vi "多参数断电保存全局变量.vi"() -> ()   [LabVIEW 2016, in "斯坦道原位多参数.lvlib"]
panel:
  in  "波特率":u32(ring)=115200 items=["9600"=9600, "19200"=19200, "115200"=115200]
  in  "传感器参数自动获取":bool=TRUE
  out "传感器参数modbus":u16[](array[numeric])
  in  "标样测试组数":dbl=1.0 caption="标样测试组数:"
  in  "水样测试组数":dbl=1.0 caption="水样测试组数:"
  in  "转刷清洗时间":dbl=30.0 caption="转刷清洗时间:"
  in  "上电初始化时间":dbl=5.0 caption="上电初始化时间:"
  in  "水样稳定时间":dbl=5.0 caption="水样稳定时间:"
  in  "ORP参数":T1
  in  "藻密度参数":T1
  in  "叶绿素参数":T1
  in  "浊度参数":T1
  in  "电导率参数":T1
  in  "溶解氧参数":T1
  in  "PH参数":T1
  in  "水温参数":T1
  in  "VISA Resource":refnum<visa-resource-name>="COM6"
  in  "运行周期":T2
  in  "质控参数设置":T3
  # "组"
  # "min"
  # "组"
  # "s"
  # "s"
  # "运行模式："
  # "质控参数设置"
  # "监测参数"
  # "水温"
  # "酸碱度"
  # "溶解氧"
  # "电导率"
  # "浊度"
  # "标样核查标准液浓度"
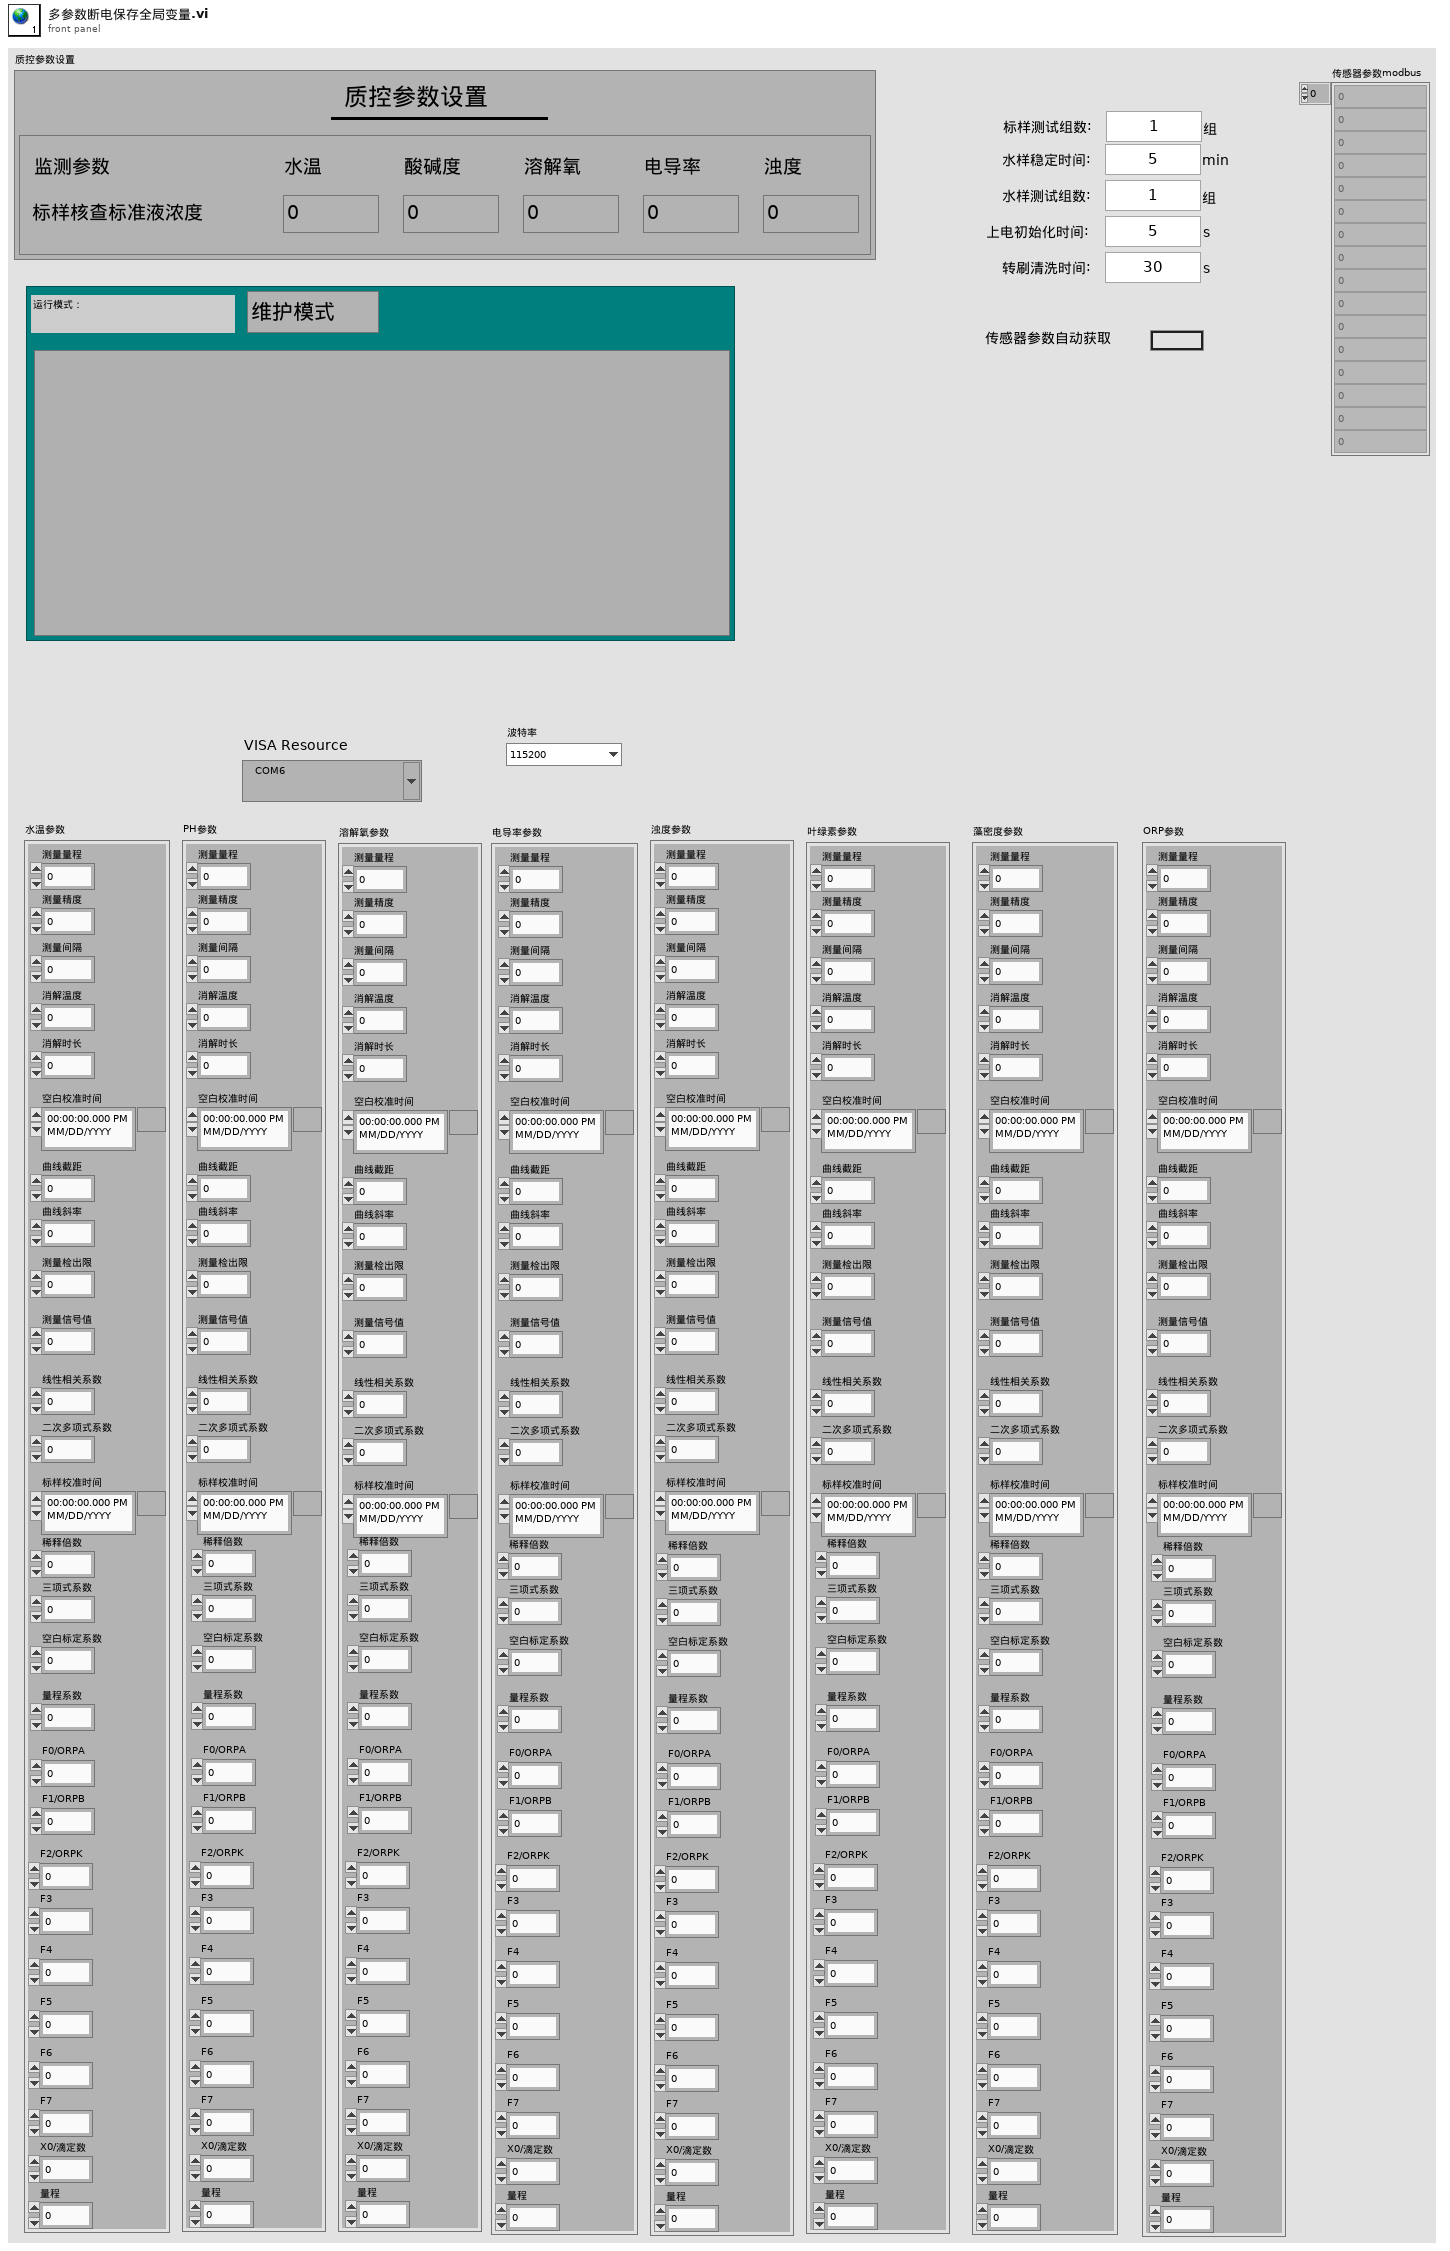
[diagram p1: front panel]
types:
  T1 = cluster{"测量量程":dbl, "测量精度":dbl, "测量间隔":dbl, "消解温度":dbl, "消解时长":dbl, "空白校准时间":timestamp, "曲线截距":dbl, "曲线斜率":dbl, "测量检出限":dbl, "测量信号值":dbl, "线性相关系数":dbl, "二次多项式系数":dbl, "标样校准时间":timestamp, "稀释倍数":dbl, "三项式系数":dbl, "空白标定系数":dbl, "量程系数":dbl, "F0/ORPA":dbl, "F1/ORPB":dbl, "F2/ORPK":dbl, "F3":dbl, "F4":dbl, "F5":dbl, "F6":dbl, "F7":dbl, "X0/滴定数":dbl, "量程":dbl}
  T2 = cluster{"运行模式":enum16{"维护模式", "常规模式", "应急模式", "质控模式"}, "24H周期设置":bool[]}
  T3 = cluster{"水温标准液标准浓度":dbl, "酸碱度标准液标准浓度":dbl, "溶解氧标准液标准浓度":dbl, "电导率标准液标准浓度":dbl, "浊度标准液标准浓度":dbl}
diagram:
